vi "Message Get Message Type.vi"(2 "Message Types":string[](array[string]), 3 "Message":string) -> (0 "Trailing text":string, 1 "Message Type":i32)   [LabVIEW 2010]
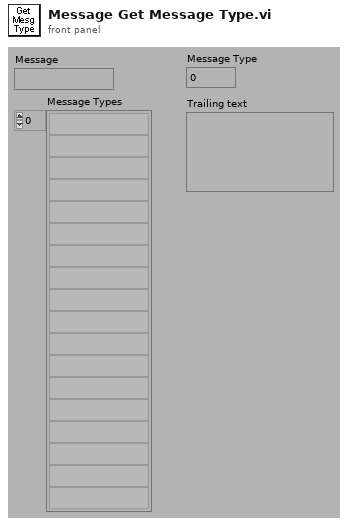
[diagram p1: front panel]
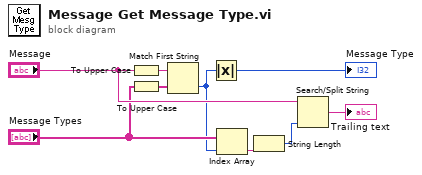
[diagram p0: block diagram]
diagram:
  n1 = To Upper Case(1:"Message") -> (0:w2:string)
  n2 = To Upper Case(1:"Message Types") -> (0:w3:string[])
  n3 = Match First String(2:w3, 3:w2) -> (0:w6:i32)  [unwired: 1 out]
  n4 = Absolute Value(x=w6) -> (abs(x)=→"Message Type":i32)
  n5 = Index Array(array="Message Types", index=w6) -> (element=w5:string)
  n6 = String Length(string=w5) -> (length=w4:i32)
  n7 = Search/Split String(string="Message", offset (0)=w4) -> (match + rest of string=→"Trailing text":string)  [unwired: 1 in, 2 out]
